vi "MF-101 PWM Push, Pull and Push Pull test with Guardian.vi"() -> ()   [LabVIEW 8.6]
uses:
  <libdir>/resource/objmgr/ueidaq.rc
  vi.lib/UeiDaq/UeiDaqConfigureTimingForSimpleIO.vi
  vi.lib/UeiDaq/UeiDaqReadOneScaledScan.vi
  vi.lib/UeiDaq/UeiDaqCreateDOIndustrialSession.vi
panel:
  out "PWM output mode":i32[](array[ring]) items=["Push", "Pull", "Push-Pull", "Off"]
  in  "PWM output mode":i32[](array[ring]) items=["Push", "Pull", "Push-Pull", "Off"]
  in  "duty cycle":dbl[](array[numeric])
  in  "stop":bool
  in  "Diagnostic Resource":string
  out "Diaganostic data ( volts )":dbl[](array[numeric]) format="%#_4g"
  out "Duty Cycle (%)":dbl
  out "Freq (Hz)":dbl format="%#_6f"
  out "PWM period (ms)":dbl
  in  "PWM duty cycle":dbl[](array[numeric])
  in  "PWM period":i32[](array[numeric])
  in  "PWM length":i32[](array[numeric])
  in  "PWM mode":i32[](array[ring]) items=["Disabled", "Soft-Start", "Soft-Stop", "Soft-start-stop", "Continuous", "Gated"]
  out "Device:Name":string
  out "PWM duty cycle":dbl[](array[numeric])
  out "PWM period":i32[](array[numeric])
  out "PWM length":i32[](array[numeric])
  out "PWM mode":i32[](array[ring]) items=["Disables", "Soft-Start", "Soft-Stop", "Soft-start-stop", "Continuous", "Gated"]
  in  "MF-101 Resource":string
  # "MF-101 PWM Push, Pull and Push/Pull Test Program with Guardian voltages"
  # "1/ Set the resource name -->"
  # "Diag ch0 = temp_aout0\nDiag ch1 =vsense_p_aout\nDiag ch2 =vsense_n_aout\nDiag ch3 = vdcp_p_aout0\nDiag ch4 =  temp_aout1\nDiag ch5 = vsense_p_aout1\nDiag ch6 = vsense_n_aout1\nDiag ch7 = vdcp_p_aout1\nDiag ch8 = adc_fet0\nDiag ch9 = adc_fet1\nDiag ch10 = adc_fet2\nDiag ch11 = adc_fet3\nDiag ch12 = adc_fet4\nDiag ch13 = adc_fet5\nDiag ch14 = adc_fet6\nDiag ch15 = adc_fet7\nDiag ch16 = adc_fet8\nDiag ch17 = adc_fet9\nDiag ch18 = adc_fet10\nDiag ch19  = adc_fet11\nDiag ch20 = adc_fet12\nDiag ch21 = adc_fet13\nDiag ch22 = adc_fet14\nDiag ch23\t= adc_fet15"
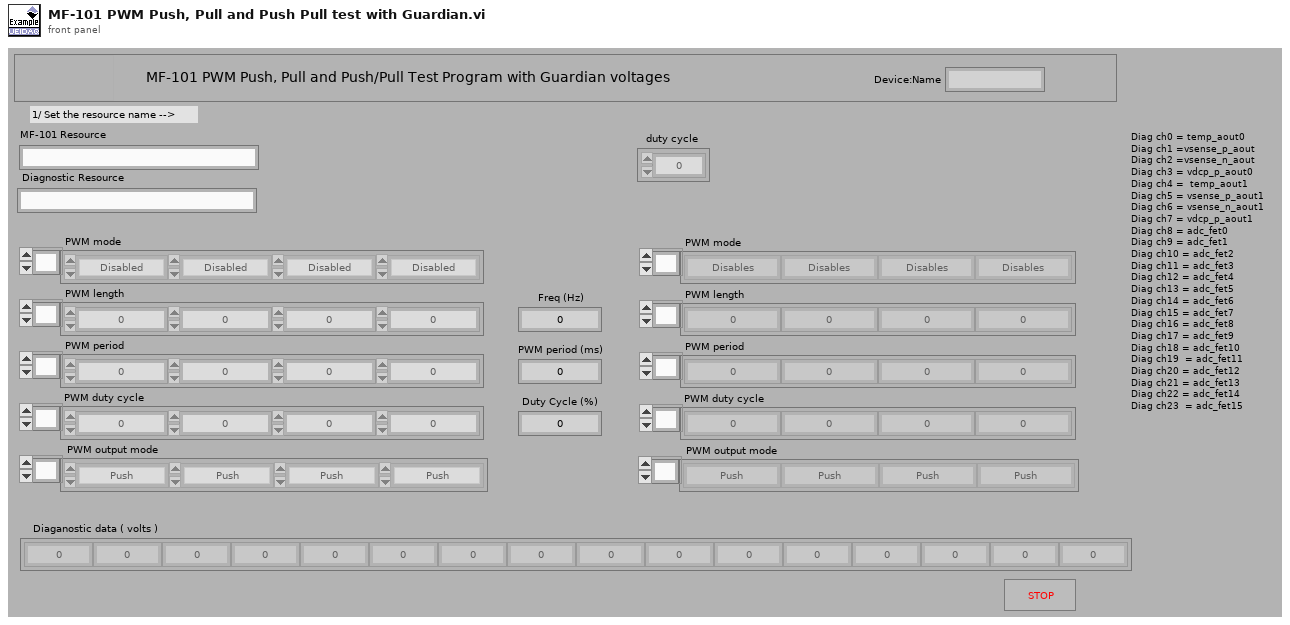
[diagram p1: front panel]
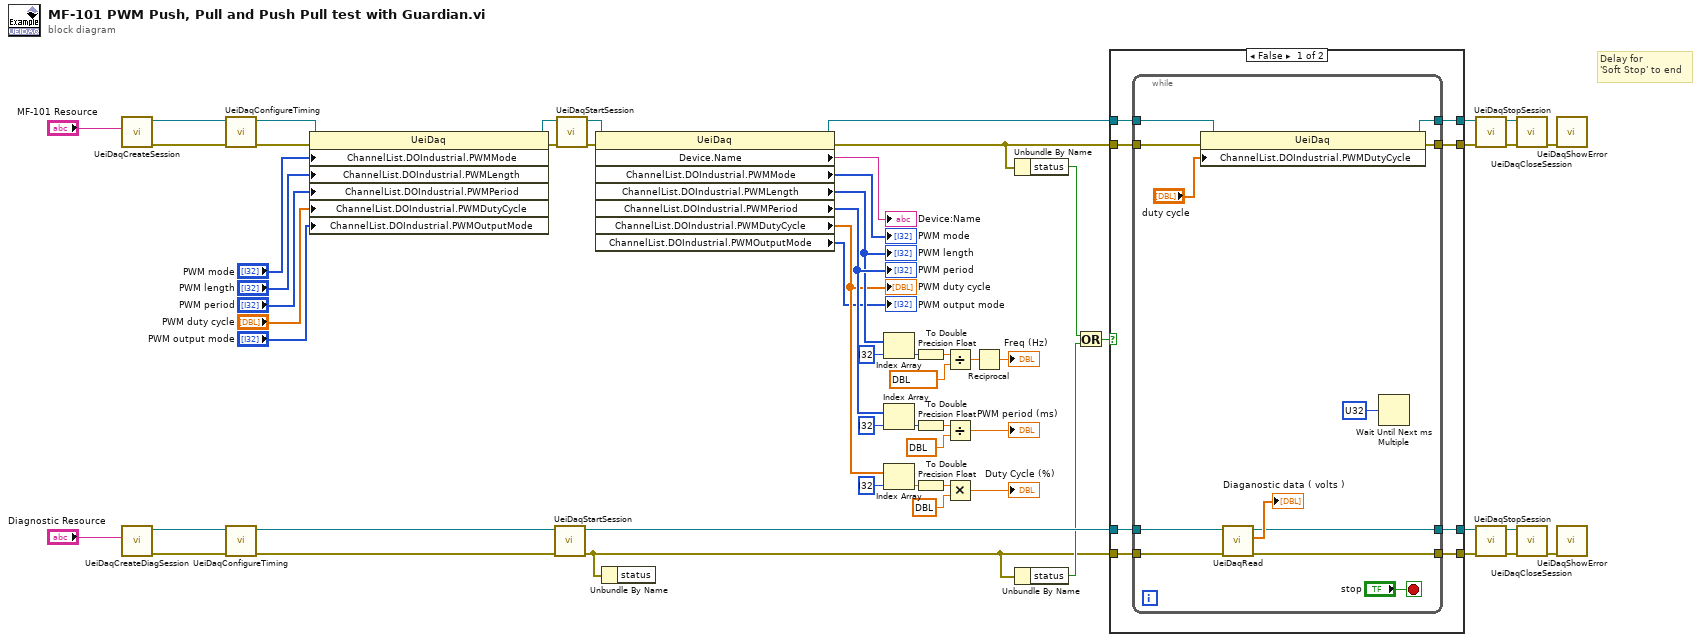
[diagram p0: block diagram]
diagram:
  # "Delay for \n'Soft Stop' to end"
  n1 = call-poly "UeiDaqCreateSession.vi"("Resource"="MF-101 Resource") -> ("error out"=w56:errorcluster, "UeiDaq Refnum Out"=w57:refnum<k20>)  [unwired: 7 in, 2 out]
  n2 = call "UeiDaqCreateDiagSession.vi"("Resource"="Diagnostic Resource") -> ("error out"=w18:errorcluster, "UeiDaq Refnum Out"=w19:refnum<k20>)  [unwired: 9 in]
  n3 = call-poly "UeiDaqConfigureTiming.vi"("error in (no error)"=w56, "UeiDaq Refnum In"=w57) -> ("error out"=w51:errorcluster, "UeiDaq Refnum Out"=w52:refnum<k20>)  [unwired: 1 in, 7 out]
  n4 = call-poly "UeiDaqConfigureTiming.vi"("error in (no error)"=w18, "UeiDaq Refnum In"=w19) -> ("error out"=w20:errorcluster, "UeiDaq Refnum Out"=w21:refnum<k20>)  [unwired: 8 out]
  n5 = property class="UeiDaq"(reference=w52, error in=w51, "ChannelList.DOIndustrial.PWMMode"="PWM mode", "ChannelList.DOIndustrial.PWMLength"="PWM length", "ChannelList.DOIndustrial.PWMPeriod"="PWM period", "ChannelList.DOIndustrial.PWMDutyCycle"="PWM duty cycle", "ChannelList.DOIndustrial.PWMOutputMode"="PWM output mode") -> (reference out=w44:refnum<k20>, error out=w43:errorcluster)
  n6 = call "UeiDaqStartSession.vi"("error in (no error)"=w20, "UeiDaq Refnum In"=w21) -> ("error out"=w8:errorcluster, "UeiDaq Refnum Out"=w16:refnum<k20>)  [unwired: 8 in]
  n7 = call "UeiDaqStartSession.vi"("error in (no error)"=w43, "UeiDaq Refnum In"=w44) -> ("error out"=w42:errorcluster, "UeiDaq Refnum Out"=w41:refnum<k20>)  [unwired: 8 in]
  n8 = property class="UeiDaq"(reference=w41, error in=w42) -> (reference out=w4:refnum<k20>, error out=w3:errorcluster, "Device.Name"=→"Device:Name":string, "ChannelList.DOIndustrial.PWMMode"=→"PWM mode":i32[], "ChannelList.DOIndustrial.PWMLength"=w35:i32[], "ChannelList.DOIndustrial.PWMPeriod"=w37:i32[], "ChannelList.DOIndustrial.PWMDutyCycle"=w22:dbl[], "ChannelList.DOIndustrial.PWMOutputMode"=→"PWM output mode":i32[])
  "PWM length" <- w35
  "PWM period" <- w37
  "PWM duty cycle" <- w22
  n9 = Unbundle By Name(w8) -> ()  [unwired: 1 out]
  n10 = Index Array(array=w35, index=i32 ?) -> (element=w34:i32)
  n11 = Index Array(array=w37, index=i32 ?) -> (element=w39:i32)
  n12 = Index Array(array=w22, index=i32 ?) -> (element=w24:dbl)
  n13 = To Double Precision Float(number=w34) -> (double precision float=w29:dbl)
  n14 = To Double Precision Float(number=w39) -> (double precision float=w32:dbl)
  n15 = To Double Precision Float(number=w24) -> (double precision float=w26:dbl)
  n16 = Divide(x=w29, y=dbl ?) -> (x/y=w28:dbl)
  n17 = Divide(x=w32, y=dbl ?) -> (x/y=→"PWM period (ms)":dbl)
  n18 = Multiply(x=w26, y=dbl ?) -> (x*y=→"Duty Cycle (%)":dbl)
  n19 = Reciprocal(x=w28) -> (1/x=→"Freq (Hz)":dbl)
  n20 = Unbundle By Name(w3) -> ("status"=w10:bool)
  n21 = Unbundle By Name(w8) -> ("status"=w9:bool)
  n22 = Or(x=w10, y=w9) -> (x .or. y?=w7:bool)
  n23 = case shown="False" w7 {
    tunnel: w3 -> [w66 w81]
    tunnel: [w65 w81] -> w1
    tunnel: w4 -> [w64 w82]
    tunnel: [w63 w82] -> w2
    tunnel: w16 -> [w62 w80]
    tunnel: w8 -> [w61 w79]
    tunnel: [w60 w80] -> w12
    tunnel: [w59 w79] -> w11
    frame #0 {
      n24 = while {
        tunnel: w66 -> [w71]
        tunnel: [w69] -> w65
        tunnel: w64 -> [w70]
        tunnel: [w68] -> w63
        tunnel: w62 -> [w78]
        tunnel: w61 -> [w77]
        tunnel: [w75] -> w59
        tunnel: [w74] -> w60
        stop <- "stop" stop-if-true
        n25 = property class="UeiDaq"(reference=w70, error in=w71, "ChannelList.DOIndustrial.PWMDutyCycle"="duty cycle") -> (reference out=w68:refnum<k20>, error out=w69:errorcluster)
        n26 = call-poly "UeiDaqRead.vi"("error in (no error)"=w77, "UeiDaq Refnum In"=w78) -> ("error out"=w75:errorcluster, "Scaled Data"=→"Diaganostic data ( volts )":dbl[], "UeiDaq Refnum Out"=w74:refnum<k20>)  [unwired: 7 in]
        n27 = Wait Until Next ms Multiple(millisecond multiple=u32 ?) -> ()  [unwired: 1 out]
      }
    }
    frame #1 {
    }
  }
  n28 = call "UeiDaqStopSession.vi"("error in (no error)"=w1, "UeiDaq Refnum In"=w2) -> ("error out"=w45:errorcluster, "UeiDaq Refnum Out"=w46:refnum<k20>)  [unwired: 8 in]
  n29 = call "UeiDaqStopSession.vi"("error in (no error)"=w11, "UeiDaq Refnum In"=w12) -> ("error out"=w15:errorcluster, "UeiDaq Refnum Out"=w14:refnum<k20>)  [unwired: 8 in]
  n30 = call "UeiDaqCloseSession.vi"("error in (no error)"=w45, "UeiDaq Refnum In"=w46) -> ("error out"=w58:errorcluster)  [unwired: 1 in, 8 out]
  n31 = call "UeiDaqCloseSession.vi"("error in (no error)"=w15, "UeiDaq Refnum In"=w14) -> ("error out"=w13:errorcluster)  [unwired: 1 in, 8 out]
  n32 = call "UeiDaqShowError.vi"("error in (no error)"=w58) -> ()  [unwired: 2 in, 9 out]
  n33 = call "UeiDaqShowError.vi"("error in (no error)"=w13) -> ()  [unwired: 2 in, 9 out]
